vi "Lookup ID.vi"(8 "error in (no error)":errorcluster, 10 "ID":string, 11 "SensorList in":refnum<class "SensorList.lvclass">) -> (0 "error out":errorcluster, 2 "Sensor":refnum<class "Sensor Config.lvclass">, 3 "SensorList out":refnum<class "SensorList.lvclass">)   [LabVIEW 2020, in "VolatusConfig.lvlib" / "SensorList.lvclass"]
uses:
  SensorList.lvclass
  C:/dev/lv20CE/relink/lv-volatus/VolatusConfig/VolatusConfigElement/VolatusConfigElement.lvclass
  Sensor/Sensor Config.lvclass
  VolatusConfigElement/VolatusConfigElement.lvclass/VolatusConfigElement.ctl
  SensorList.lvclass/SensorList.ctl
  VolatusConfigElement/VolatusConfigElement.lvclass
  lv-cdm/CDM-Config/Config Element/Config Element.lvclass
  C:/dev/lv20CE/relink/lv-volatus/VolatusConfig/SensorList/SensorList.lvclass
  C:/dev/lv20CE/relink/lv-volatus/VolatusConfig/Sensor/Sensor Config.lvclass
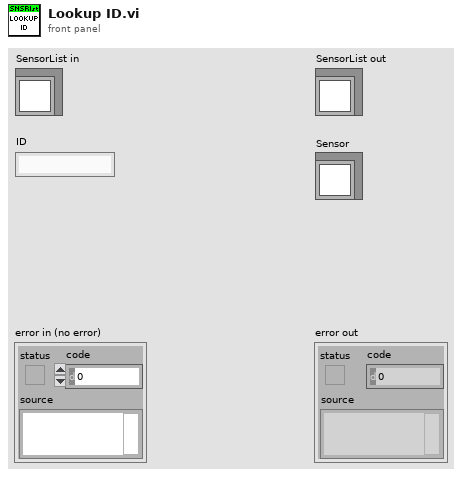
[diagram p1: front panel]
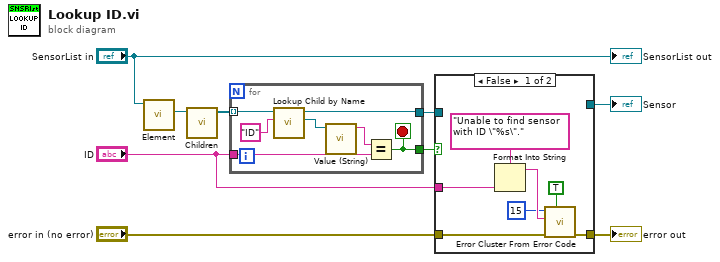
[diagram p0: block diagram]
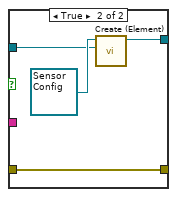
[diagram p2: hidden frame]
diagram:
  n1 = call "Element.vi"("VolatusConfigElement in"="SensorList in") -> ("Element"=w8:refnum<class "Config Element.lvclass">)  [unwired: 9 in, 1 out]
  n2 = call "Children.vi"("Config Element in"=w8) -> ("Elements"=w7:refnum<class "Config Element.lvclass">[])  [unwired: 9 in, 1 out]
  n3 = for {
    tunnel: w7 -> [w12] mode=indexing
    tunnel: "ID" -> [w11]
    tunnel: [w13] -> w6
    tunnel: [w10] -> w5
    stop <- w10 stop-if-true
    n4 = call "Lookup Child by Name.vi"("Name"="ID", "Config Element in"=w12) -> ("Child"=w15:refnum<class "Config Element.lvclass">, "Config Element out"=w13:refnum<class "Config Element.lvclass">)  [unwired: 6 in, 2 out]
    n5 = call "Value (String).vi"("Config Element in"=w15) -> ("String Value"=w14:string)  [unwired: 9 in, 1 out]
    n6 = Equal?(x=w14, y=w11) -> (x = y?=w10:bool)
  }
  n7 = case shown="False" w5 {
    tunnel: w6 -> [_ w25]
    tunnel: "error in (no error)" -> [w23 w27]
    tunnel: "ID" -> [w20 _]
    tunnel: [w22 w27] -> w2
    tunnel: [_ w24] -> w1
    frame False {
      n8 = Format Into String(format string="Unable to find sensor with ID \"%s\".", w20) -> (resulting string=w18:string)  [unwired: 2 in, 1 out]
      n9 = call <vilib>:"Error Cluster From Error Code.vi"("show call chain? (False)"=TRUE, "error in (no error)"=w23, "error message (\"\")"=w18, "error code (0)"=15) -> ("error out"=w22:errorcluster)  [unwired: 5 in]
    }
    frame True {
      n10 = call "Create (Element).vi"("Element"=w25, "VolatusConfigElement in"=refnum<class "Sensor Config.lvclass"> refnum ("VolatusConfig.lvlib:Sensor")) -> ("VolatusConfigElement out"=w24:refnum<class "Sensor Config.lvclass">)  [unwired: 8 in, 1 out]
    }
  }
  "error out" <- w2
  "Sensor" <- w1
  "SensorList out" <- "SensorList in"
